vi "EdgeDetection.vi"() -> ()   [LabVIEW 2017]
uses:
  <vilib>/LabVIEW Interface for Arduino/Type Defs/Board Type.ctl
  <vilib>/LabVIEW Interface for Arduino/Type Defs/Connection Type.ctl
  <vilib>/LabVIEW Interface for Arduino/Type Defs/Pin Mode.ctl
  <vilib>/LabVIEW Interface for Arduino/LabVIEW Interface for Arduino.lvlib
panel:
  in  "VISA resource name 2":refnum<visa-resource-name>="COM1"
  in  "Baud Rate 2":u32=115200
  in  "Connection Type":T1
  in  "Board Type":T2
  out "Digital Waveform":dbl(graph)
  out "Pulse Count":dbl
  out "E-STOP":bool
  out "Edge Detection":bool
  in  "Program Stop":bool
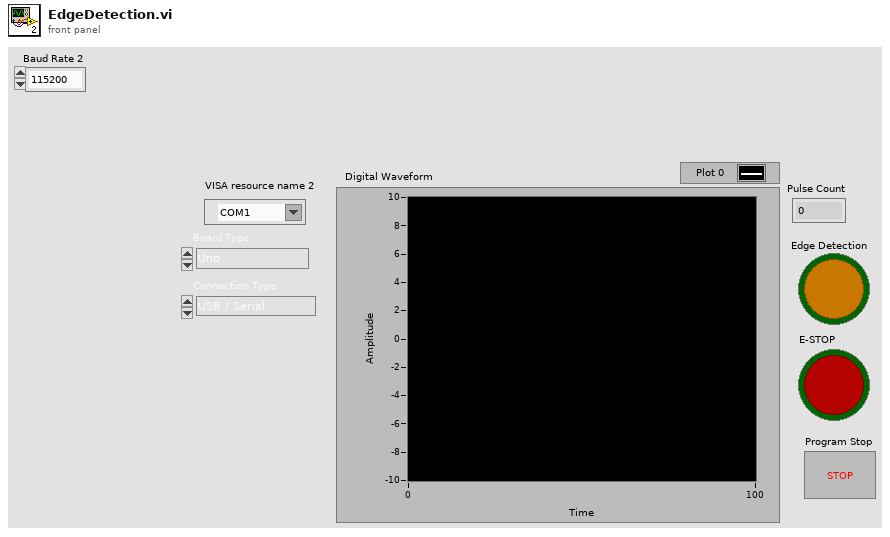
[diagram p1: front panel]
types:
  T1 = typedef "LabVIEW Interface for Arduino.lvlib/Connection Type.ctl" = enum8{"USB / Serial", "XBEE", "BlueSmirf (Bluetooth)"}
  T2 = typedef "LabVIEW Interface for Arduino.lvlib/Board Type.ctl" = enum16{"Uno", "Dimuelanove w/Atmega 328", "Mega 2560"}
  T3 = typedef "LabVIEW Interface for Arduino.lvlib/Pin Mode.ctl" = enum8{"Input", "Output"}
  T4 = typedef "LabVIEW Interface for Arduino.lvlib/Arduino Resource.ctl" = cluster{"VISA resource":refnum<visa-resource-name>, "Board Type":T2, "Connection Type":enum8{"USB / Serial"}, "Bytes Per Packet (15)":u8}
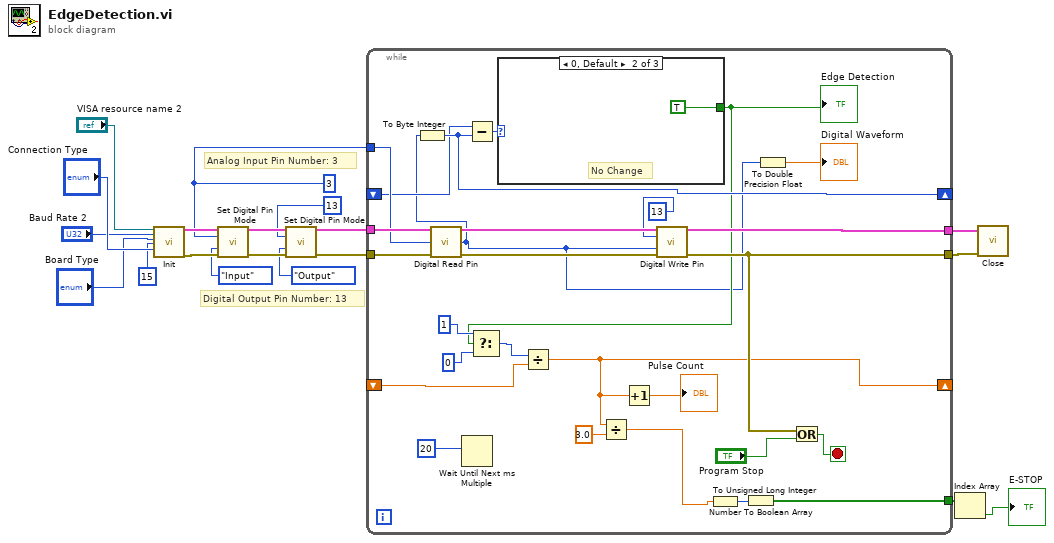
[diagram p0: block diagram]
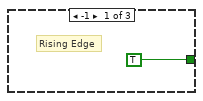
[diagram p2: hidden frame]
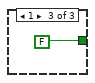
[diagram p3: hidden frame]
diagram:
  w8 = u8 3 ("Digital I/O Pin")
  # "Digital Output Pin Number: 13"
  # "Analog Input Pin Number: 3"
  n1 = call <vilib>:"Init.vi"("VISA resource"="VISA resource name 2", "Baud Rate (115200)"="Baud Rate 2", "Board Type (Uno)"="Board Type", "Bytes Per Packet (15)"=u8 15, "Connection Type (USB/Serial)"="Connection Type") -> ("Arduino Resource"=w19:T4, "error out"=w18:errorcluster)  [unwired: 13 in]
  n2 = call <vilib>:"Set Digital Pin Mode.vi"("Arduino Resource"=w19, "Digital I/O Pin"=w8, "Pin Mode (Input)"=Pin_Mode."Input", "error in"=w18) -> ("Arduino Resource"=w16:T4, "error out"=w15:errorcluster)  [unwired: 10 in]
  n3 = call <vilib>:"Set Digital Pin Mode.vi"("Arduino Resource"=w16, "Digital I/O Pin"=u8 13, "Pin Mode (Input)"=Pin_Mode."Output", "error in"=w15) -> ("Arduino Resource"=w11:T4, "error out"=w12:errorcluster)  [unwired: 10 in]
  n4 = while {
    tunnel: w8 -> [w37]
    tunnel: w12 -> [w44]
    tunnel: w11 -> [w45]
    tunnel: [w25] -> w10
    tunnel: [w41] -> w9
    shift-right: [w35] -> _
    shift-left: _ -> [w34]
    shift-right: [w20] -> _
    shift-left: _ -> [w30]
    tunnel: [w28] -> w7
    stop <- w40 stop-if-true
    n5 = call <vilib>:"Digital Read Pin.vi"("Arduino Resource"=w45, "Digital I/O Pin (0)"=w37, "error in"=w44) -> ("Arduino Resource"=w42:T4, "Value"=w22:u8, "error out"=w43:errorcluster)  [unwired: 10 in]
    n6 = To Byte Integer(number=w22) -> (8bit integer=w35:i8)
    n7 = Wait Until Next ms Multiple(millisecond multiple=u32 20) -> ()  [unwired: 1 out]
    n8 = Subtract(x=w34, y=w35) -> (x-y=w46:i8)
    n9 = case shown="0, Default" w46 {
      tunnel: [TRUE ("Boolean") TRUE ("Boolean") FALSE ("Boolean")] -> w24
      frame -1 {
        # "Rising Edge"
      }
      frame 0, Default {
        # "No Change"
      }
      frame 1 {
      }
    }
    "Edge Detection" <- w24
    n10 = Select(t=1, s=w24, f=0) -> (s? t:f=w31:i32)
    n11 = Divide(x=w31, y=w30) -> (x/y=w20:dbl)
    n12 = Divide(x=w20, y=3.0) -> (x/y=w26:dbl)
    n13 = Increment(x=w20) -> (x+1=→"Pulse Count":dbl)
    n14 = call <vilib>:"Digital Write Pin.vi"("Arduino Resource"=w42, "Digital I/O Pin (0)"=u8 13, "Value (0)"=w22, "error in"=w43) -> ("Arduino Resource"=w25:T4, "error out"=w41:errorcluster)  [unwired: 10 in]
    n15 = To Unsigned Long Integer(number=w26) -> (unsigned 32bit integer=w29:u32)
    n16 = Number To Boolean Array(number=w29) -> (Boolean array=w28:bool[])
    n17 = To Double Precision Float(number=w22) -> (double precision float=→"Digital Waveform":dbl)
    n18 = Or(x=w41, y="Program Stop") -> (x .or. y?=w40:bool)
  }
  n19 = Index Array(array=w7) -> (element=→"E-STOP":bool)  [unwired: 1 in]
  n20 = call <vilib>:"Close.vi"("Arduino Resource"=w10, "error in"=w9) -> ()  [unwired: 13 in, 1 out]
